vi "水质测量数据table定义.vi"(5 "数据标记表":string(combo)="N", 7 "table 输入":string, 9 "SN":string, 10 "测量模式":T2(ring)=enum."水样测试", 11 "data":T1 {"单位" items=["ug/L", "mg/L", "ppm", "mg/m3", "cm", "ppb", "ug/m3", "%", "nmol/mol", "umol/mol", "MPN/L", "MPN/100ml", "ng/m3", "NTU", "无量纲", "ms/cm", "us/cm"]}) -> (1 "table 输出":string, 2 "columns":string[](array[string]), 3 "data输出":T3)   [LabVIEW 2016, in "斯坦道CODMn新电路板.lvlib"]
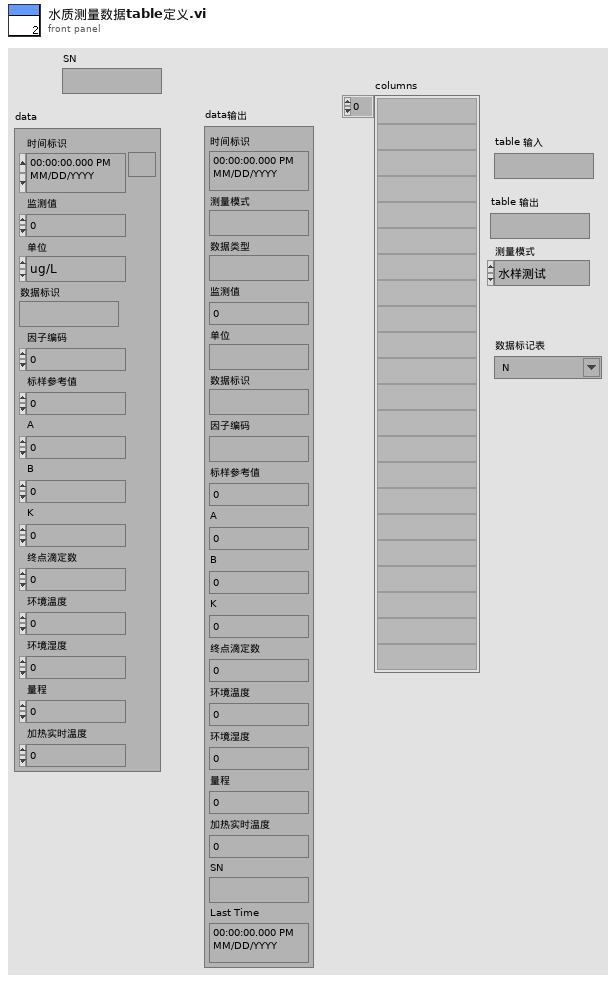
[diagram p1: front panel]
types:
  T1 = cluster{"时间标识":timestamp, "监测值":sgl, "单位":u16, "数据标识":string, "因子编码":u32, "标样参考值":sgl, "A":sgl, "B":sgl, "K":sgl, "终点滴定数":sgl, "环境温度":sgl, "环境湿度":sgl, "量程":sgl, "加热实时温度":sgl}
  T2 = enum16{"维护数据", "水样测试", "标样核查", "零点核查", "跨度核查", "空白测试", "平行样测试", "加标回收", "空白校准", "标样校准", "初始化（清洗）"}
  T3 = cluster{"时间标识":timestamp, "测量模式":string, "数据类型":string, "监测值":sgl, "单位":string, "数据标识":string, "因子编码":string, "标样参考值":sgl, "A":sgl, "B":sgl, "K":sgl, "终点滴定数":sgl, "环境温度":sgl, "环境湿度":sgl, "量程":sgl, "加热实时温度":sgl, "SN":string, "Last Time":timestamp}
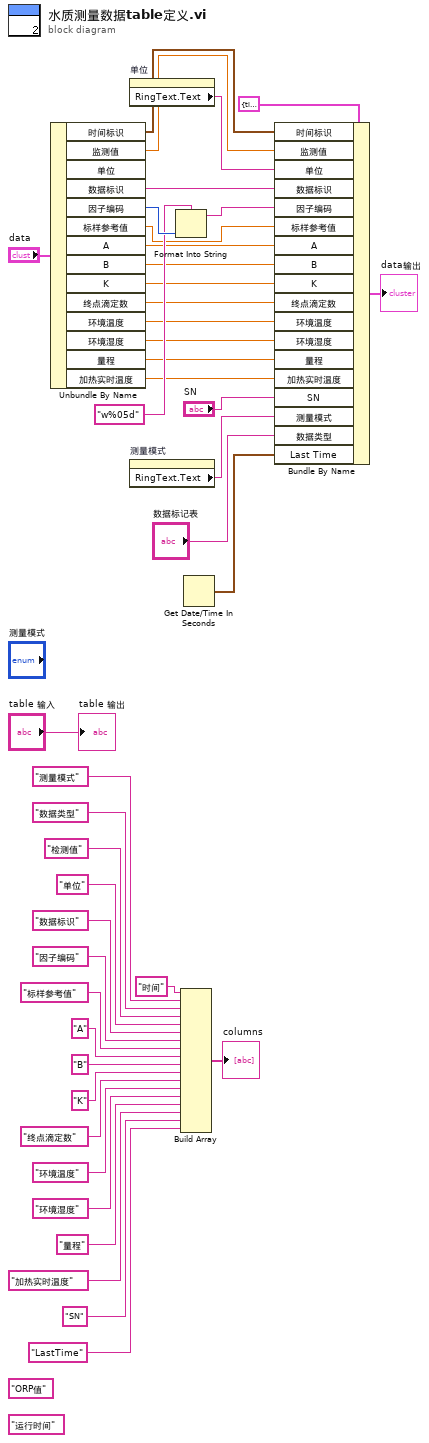
[diagram p0: block diagram]
diagram:
  (unwired) "ORP值"
  (unwired) "运行时间"
  n1 = Unbundle By Name("data") -> ("时间标识"=w30:timestamp, "监测值"=w29:sgl, "数据标识"=w28:string, "因子编码"=w33:u32, "标样参考值"=w26:sgl, "A"=w16:sgl, "B"=w15:sgl, "K"=w14:sgl, "终点滴定数"=w13:sgl, "环境温度"=w12:sgl, "环境湿度"=w11:sgl, "量程"=w10:sgl, "加热实时温度"=w9:sgl)  [unwired: 1 out]
  n2 = property on="单位" class="Ring (严格)"() -> ("RingText.Text"=w17:string)  [unwired: 2 in, 2 out]
  n3 = property on="测量模式" class="Enum (严格)"() -> ("RingText.Text"=w6:string)  [unwired: 2 in, 2 out]
  n4 = Format Into String(format string="w%05d" ("格式字符串"), w33) -> (resulting string=w31:string)  [unwired: 2 in, 1 out]
  n5 = Build Array("时间", "测量模式", "数据类型", "检测值", "单位", "数据标识", "因子编码", "标样参考值", "A", "B", "K", "终点滴定数", "环境温度", "环境湿度", "量程", "加热实时温度", "SN", "LastTime") -> (→"columns":string[])
  n6 = Get Date/Time In Seconds() -> (seconds since 1Jan1904=w4:timestamp)
  n7 = Bundle By Name(cluster=T3 {"时间标识"=timestamp(0 s since 1904-01-01), "测量模式"="", "数据类型"="", "监测值"=0.0, "单位"="", "数据标识"="", "因子编码"="", "标样参考值"=0.0, "A"=0.0, "B"=0.0, "K"=0.0, "终点滴定数"=0.0, "环境温度"=0.0, "环境湿度"=0.0, "量程"=0.0, "加热实时温度"=0.0, "SN"="", "Last Time"=timestamp(0 s since 1904-01-01)} ("data输出"), "时间标识"=w30, "监测值"=w29, "单位"=w17, "数据标识"=w28, "因子编码"=w31, "标样参考值"=w26, "A"=w16, "B"=w15, "K"=w14, "终点滴定数"=w13, "环境温度"=w12, "环境湿度"=w11, "量程"=w10, "加热实时温度"=w9, "SN"="SN", "测量模式"=w6, "数据类型"="数据标记表", "Last Time"=w4) -> (→"data输出":T3)
  "table 输出" <- "table 输入"
